vi "Get Devices.vi"(8 "error in (no error)":errorcluster) -> (0 "error out":errorcluster, 2 "Device Names":string[](array[string]))   [LabVIEW 2020, in "MIDIllan.lvlib" / "midi in.lvclass"]
uses:
  midi in.lvclass
  midi in.lvclass/midi in.ctl
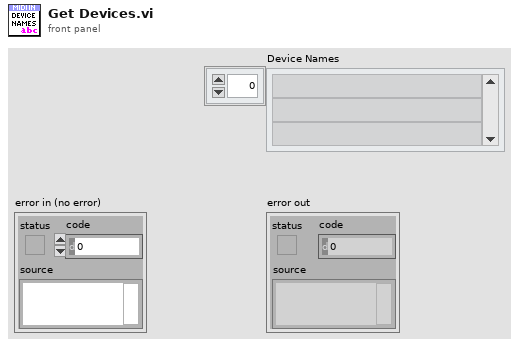
[diagram p1: front panel]
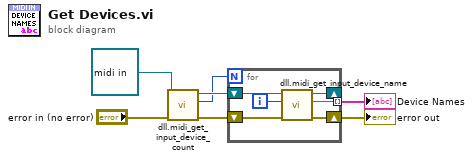
[diagram p0: block diagram]
diagram:
  n1 = call "dll.midi_get_input_device_count.vi"("error in (no error)"="error in (no error)", "LabVIEW-MIDI-XPLAT in"=refnum<class "midi in.lvclass"> refnum) -> ("error out"=w5:errorcluster, "device count"=w6:i32, "LabVIEW-MIDI-XPLAT out"=w7:refnum<class "midi in.lvclass">)  [unwired: 7 in]
  n2 = for {
    N: w6 -> [_]
    shift-right: [w10] -> w3
    shift-left: w5 -> [w11]
    tunnel: [w9] -> w2 mode=indexing
    shift-right: [w8] -> _
    shift-left: w7 -> [w13]
    i -> [w12]
    n3 = call "dll.midi_get_input_device_name.vi"("error in (no error)"=w11, "Device Index"=w12, "LabVIEW-MIDI-XPLAT in"=w13) -> ("error out"=w10:errorcluster, "Device Names"=w9:string, "LabVIEW-MIDI-XPLAT out"=w8:refnum<class "midi in.lvclass">)  [unwired: 6 in]
  }
  "error out" <- w3
  "Device Names" <- w2
